vi "Delete DB data.vi"(6 "index":i32, 8 "error in (no error)":errorcluster caption="错误输入（无错误）", 9 "code":string, 10 "table":string, 11 "Connncet State":T1) -> (0 "error out":errorcluster caption="错误输出", 3 "Connect State":T1)   [LabVIEW 2014]
uses:
  Ctr/Constr.ctl
  <vilib>/addons/database/Connection.llb/Conn ObjectReference.ctl
  <vilib>/addons/database/NI_Database_API.lvlib
  Ctr/Conneect State.ctl
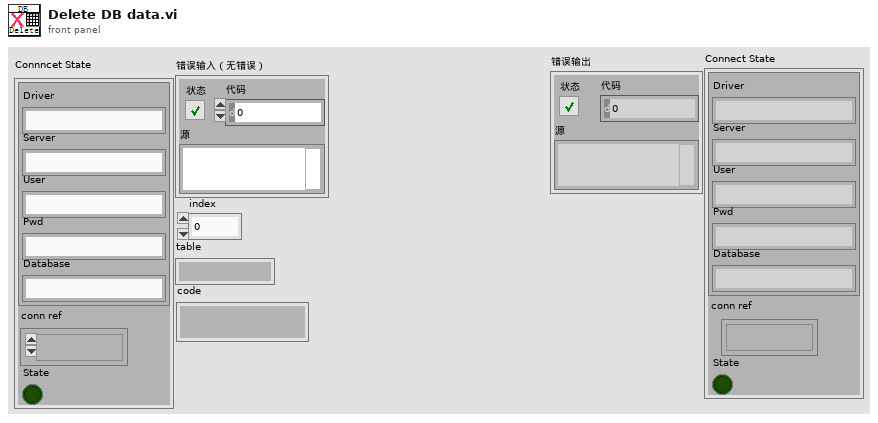
[diagram p1: front panel]
types:
  T1 = typedef "Conneect State.ctl" = cluster{"Constr":T2, "conn ref":T3, "State":bool}
  T2 = typedef "Constr.ctl" = cluster{"Driver":string, "Server":string, "User":string, "Pwd":string, "Database":string}
  T3 = typedef "NI_Database_API.lvlib/Conn ObjectReference.ctl" = refnum<k1>
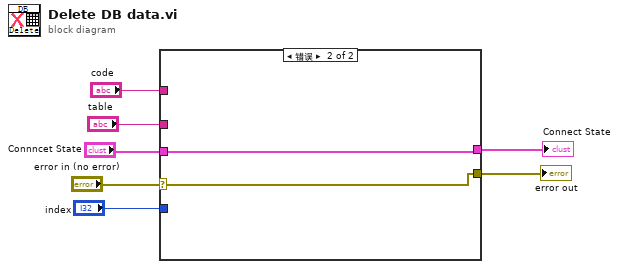
[diagram p0: block diagram]
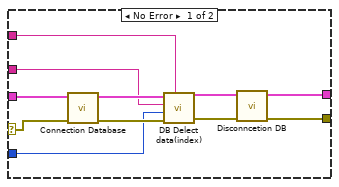
[diagram p2: hidden frame]
diagram:
  n1 = case shown="错误" "error in (no error)" {
    selector: "error in (no error)" -> [w8 w19]
    tunnel: "Connncet State" -> [w18 w20]
    tunnel: "index" -> [w15 _]
    tunnel: "table" -> [w14 _]
    tunnel: "code" -> [w13 _]
    tunnel: [w10 w19] -> w3
    tunnel: [w9 w20] -> w2
    frame No Error {
      n2 = call "Connection Database.vi"("error in (no error)"=w8, "Connncet State"=w18) -> ("error out"=w17:errorcluster, "Connncet State out"=w16:T1)  [unwired: 8 in]
      n3 = call "DB Delect data(index).vi"("code"=w13, "error in (no error)"=w17, "index"=w15, "table"=w14, "Connncet State"=w16) -> ("error out"=w12:errorcluster, "Connncet State out"=w11:T1)  [unwired: 4 in, 1 out]
      n4 = call "Disconncetion DB.vi"("error in (no error)"=w12, "Connncet State"=w11) -> ("error out"=w10:errorcluster, "Connect State"=w9:T1)  [unwired: 8 in]
    }
    frame Error {
    }
  }
  "error out" <- w3
  "Connect State" <- w2
